vi "FTW-Endpoint-CreateReader.vi"(0 "FTW-Endpoint In":refnum<class "FTW-Endpoint.lvclass">, 5 "Address":string, 11 "error in":errorcluster) -> (4 "FTW-Endpoint Out":refnum<class "FTW-Endpoint.lvclass">, 6 "Actual Address":string, 15 "error out":errorcluster)   [LabVIEW 2013, in "FTW-Endpoint.lvclass"]
uses:
  FTW-Endpoint.lvclass
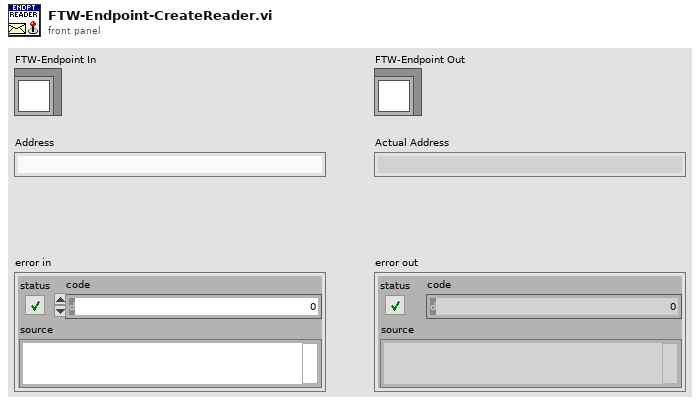
[diagram p1: front panel]
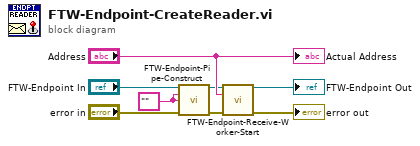
[diagram p0: block diagram]
diagram:
  w1 = "" ("empty string")
  n1 = call-dynamic "FTW-Endpoint-Pipe-Construct.vi"("FTW Endpoint"="FTW-Endpoint In", "Address"=w1, "Requested Identity"=w1, "error in"="error in") -> ("FTW Endpoint out"=w2:refnum<class "FTW-Endpoint.lvclass">, "error out"=w3:errorcluster)  [unwired: 9 in, 1 out]
  n2 = call-dynamic "FTW-Endpoint-Receive-Worker-Start.vi"("FTW-Endpoint In"=w2, "Endpoint Address"="Address", "error in"=w3) -> ("FTW-Endpoint Out"=→"FTW-Endpoint Out":refnum<class "FTW-Endpoint.lvclass">, "error out"=→"error out":errorcluster)  [unwired: 11 in]
  "Actual Address" <- "Address"
